vi "Read Analogue.vi"(8 "error in (no error)":errorcluster, 11 "niPower in":refnum<class "NI DC Power.lvclass">) -> (0 "error out":errorcluster, 2 "Waveforms":waveform(dbl)[](array[waveform]), 3 "niPower out":refnum<class "NI DC Power.lvclass">)   [LabVIEW 2025, in "Power Supply.lvlib" / "NI DC Power.lvclass"]
uses:
  NI DC Power.lvclass
  NI DC Power.lvclass/NI DC Power.ctl
  <vilib>/Analysis/baseanly.llb/Mean (DBL).vi
  <vilib>/Analysis/NI_AALBase.lvlib
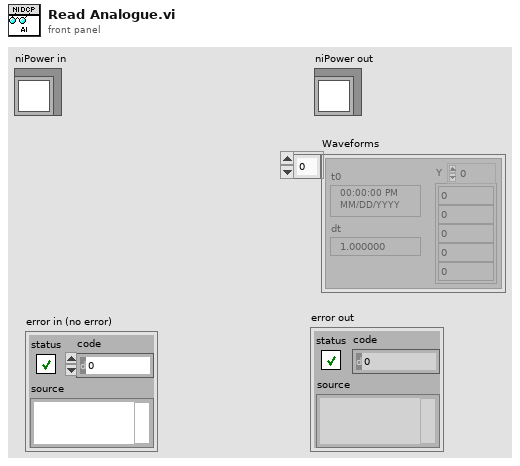
[diagram p1: front panel]
types:
  T1 = typedef "Abstract Engine.lvlibp/Abstract Instrument.lvclass/Channel.ctl" = cluster{"Alias":string, "DataType":enum16{"Anaolg Input", "Waveform"}, "Unit":enum16{"---", "V", "A", "Ohm", "Hz", "uF", "degC", "deg"}, "Upper limit":dbl, "Lower limit":dbl, "Measurement":variant}
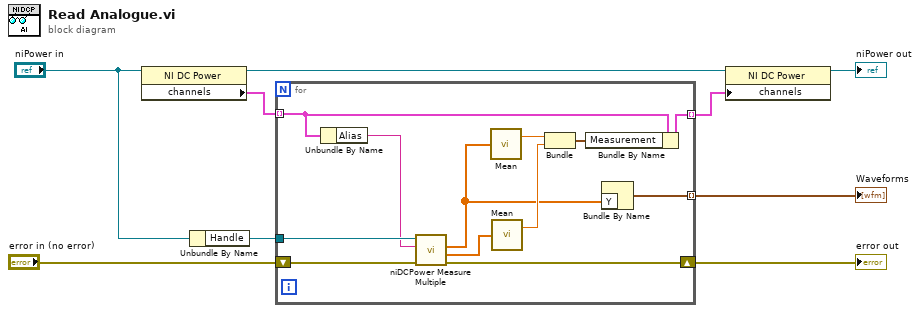
[diagram p0: block diagram]
diagram:
  n1 = property class="NI DC Power"(reference="niPower in") -> (reference out=w5:refnum<class "NI DC Power.lvclass">, "channels"=w3:T1[])  [unwired: 1 in, 1 out]
  n2 = Unbundle By Name("niPower in") -> ("Handle"=w6:refnum<k15>)
  n3 = for {
    tunnel: w6 -> [w20]
    shift-right: [w19] -> w7
    shift-left: "error in (no error)" -> [w21]
    tunnel: w3 -> [w12] mode=indexing
    tunnel: [w14] -> w2 mode=indexing
    tunnel: [w10] -> w1 mode=indexing
    n4 = Unbundle By Name(w12) -> ("Alias"=w15:string)
    n5 = call <instrlib>:"niDCPower Measure Multiple.vi"("error in (no error)"=w21, "channel name"=w15, "instrument handle"=w20) -> ("error out"=w19:errorcluster, "current measurements"=w18:dbl[], "voltage measurements"=w11:dbl[])  [unwired: 5 in, 1 out]
    n6 = call-poly <vilib>:"Mean.vi"("X"=w11) -> ("mean"=w13:dbl)  [unwired: 1 out]
    n7 = call-poly <vilib>:"Mean.vi"("X"=w18) -> ("mean"=w17:dbl)  [unwired: 1 out]
    n8 = Bundle("mean"=w13, "mean"=w17) -> (w16:cluster{"mean":dbl, "mean":dbl})  [unwired: 1 in]
    n9 = Bundle By Name(cluster=w12, "Measurement"=w16) -> (w14:T1)
    n10 = Bundle By Name("Y"=w11) -> (w10:waveform(dbl))  [unwired: 1 in]
  }
  "error out" <- w7
  "Waveforms" <- w1
  n11 = property class="NI DC Power"(reference=w5, "channels"=w2) -> (reference out=→"niPower out":refnum<class "NI DC Power.lvclass">)  [unwired: 1 in, 1 out]
